vi "ShiftRegisterV1FInal.vi"() -> ()   [LabVIEW 2020]
panel:
  out "x+1":i32
  in  "Stop Button":bool
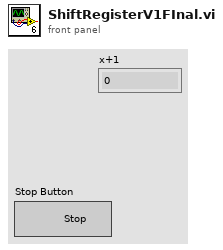
[diagram p1: front panel]
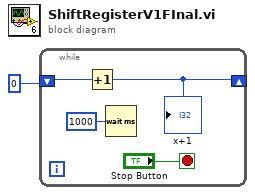
[diagram p0: block diagram]
diagram:
  n1 = while {
    shift-right: [w2] -> _
    shift-left: 0 -> [w3]
    stop <- "Stop Button" stop-if-true
    n2 = Increment(x=w3) -> (x+1=w2:i32)
    "x+1" <- w2
    n3 = Wait (ms)(milliseconds to wait=u32 1000) -> ()  [unwired: 1 out]
  }
